vi "manual_control_motors.vi"() -> ()   [LabVIEW 2017]
uses:
  <vilib>/myRIO/Common/Instrument Driver Framework/myRIO v1.0/UART/vis/myRIO v1.0 Close UART.vi
  <vilib>/myRIO/Common/Instrument Driver Framework/Utilities/vis/FPGA Ref Manager.vi
  <vilib>/myRIO/Common/Instrument Driver Framework/myRIO v1.0/myRIO v1.0 Reset FPGA.vi
  <vilib>/myRIO/Common/Instrument Driver Framework/myRIO v1.0/IRQ/vis/myRIO v1.0 IRQ Info FGV.vi
  <vilib>/myRIO/Common/Instrument Driver Framework/myRIO v1.0/IRQ/vis/myRIO v1.0 Timer IRQ Info FGV.vi
  <vilib>/myRIO/Common/Instrument Driver Framework/myRIO v1.0/IRQ/vis/myRIO v1.0 ISR Agent.vi
  <vilib>/myRIO/Instrument Drivers/Utilities/Utilities.lvlib
panel:
  in  "Speed A":dbl(slide)=-0.016713091922005565 scale=-10.0..10.0
  out "PID A":cluster{"Setpoint":dbl, "dx/dt":dbl}(graph)
  out "PID B":cluster{"Setpoint":dbl, "dx/dt":dbl}(graph)
  in  "stop":bool
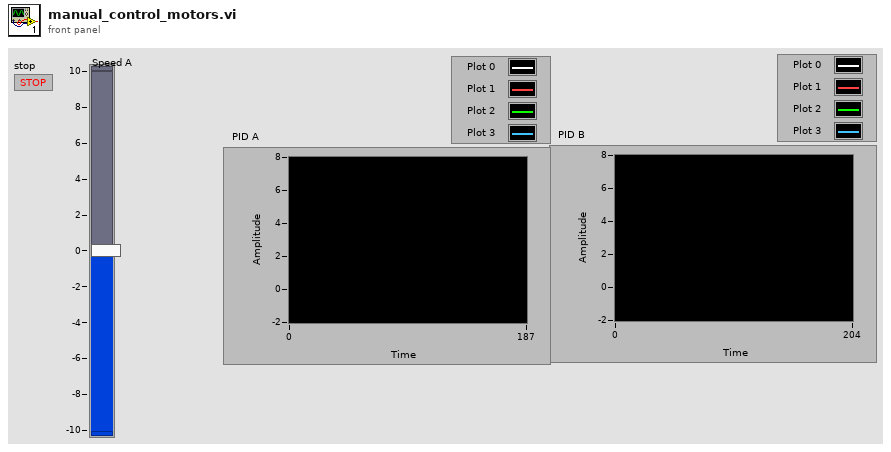
[diagram p1: front panel]
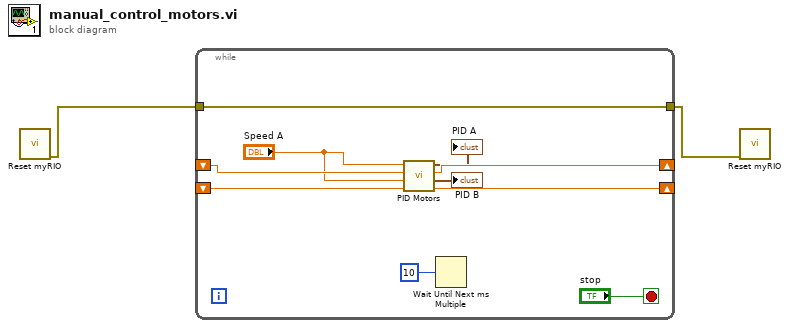
[diagram p0: block diagram]
diagram:
  n1 = call <vilib>:"Reset myRIO.vi"() -> ("error out"=w2:errorcluster)  [unwired: 11 in]
  n2 = while {
    shift-right: [w10] -> _
    shift-left: _ -> [w7]
    shift-right: [w11] -> _
    shift-left: _ -> [w6]
    tunnel: w2 -> [w4]
    tunnel: [w4] -> w1
    stop <- "stop" stop-if-true
    n3 = call "PID Motors.vi"("input B"=w7, "Speed B"="Speed A", "input A"=w6, "Speed A"="Speed A") -> ("output B"=w10:dbl, "PID B"=→"PID B":cluster{"Setpoint":dbl, "dx/dt":dbl}, "output A"=w11:dbl, "PID A"=→"PID A":cluster{"Setpoint":dbl, "dx/dt":dbl})
    n4 = Wait Until Next ms Multiple(millisecond multiple=u32 10) -> ()  [unwired: 1 out]
  }
  n5 = call <vilib>:"Reset myRIO.vi"("error in (no error)"=w1) -> ()  [unwired: 10 in, 1 out]
